vi "Achsenabschnitt berechnen.vi"(9 "Achsenabschnitt":sgl, 10 "Steigung":sgl, 11 "xmin":sgl[](array[numeric])) -> (1 "Intercept":dbl)   [LabVIEW 2020, in "Linearisierung v2.lvlib" / "Linearity verification 1065-307.lvlib"]
doc: "Berechnung des Achsenabschnitts lt. EPA 1065.307 Tab.1"
uses:
  Linearity verification 1065-307.lvlib
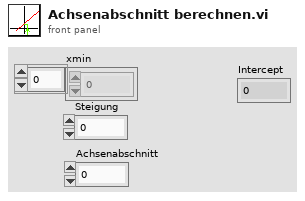
[diagram p1: front panel]
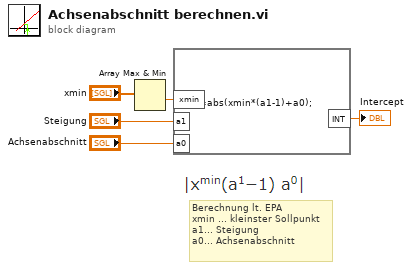
[diagram p0: block diagram]
diagram:
  # "Berechnung lt. EPA\nxmin ... kleinster Sollpunkt\na1... Steigung\na0... Achsenabschnitt"
  n1 = Array Max & Min(array="xmin") -> (min value=w1:sgl)  [unwired: 3 out]
  n2 = formula code="INT=abs(xmin*(a1-1)+a0);"("xmin"=w1, "a1"="Steigung", "a0"="Achsenabschnitt") -> ("INT"=→"Intercept":dbl)
